vi "prova1.vi"() -> ()   [LabVIEW 2020]
uses:
  <vilib>/Analysis/6fits.llb/Confidence Interval (Linear).vi
  <vilib>/Utility/file.llb/Write Delimited Spreadsheet (DBL).vi
  <vilib>/Analysis/NI_AALPro.lvlib
panel:
  out "delta R (Ohm)":dbl
  out "R (Ohm)":dbl
  out "delta q":dbl
  out "q":dbl
  out "delta m":dbl
  out "m":dbl
  out "Fit i-V":cluster{dbl[], dbl[]}[](graph)
  out "i-V":cluster{dbl[], dbl[]}(graph)
  in  "Device Name":tag
  in  "N step":dbl
  in  "Vmin":dbl
  in  "Vmax":dbl
  in  "Esci":bool
  in  "Salva Dati":bool
  in  "Misura":bool
  in  "Analizza":bool
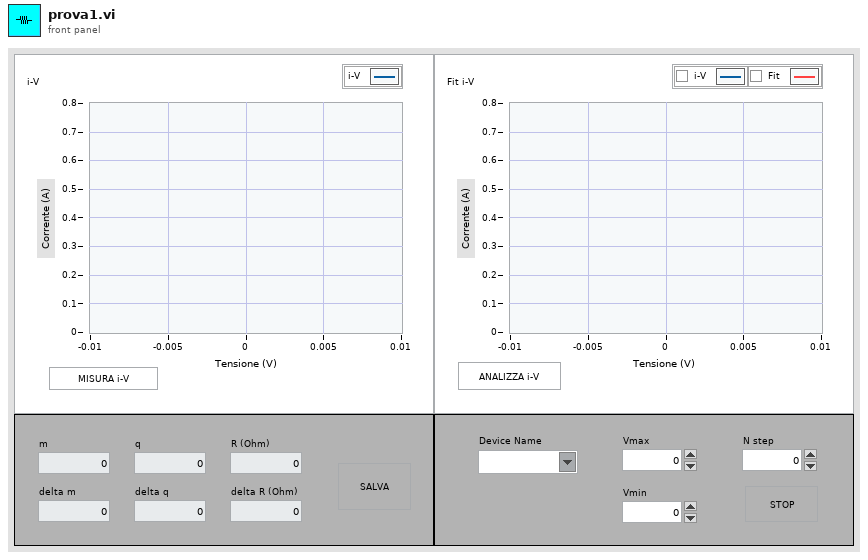
[diagram p1: front panel]
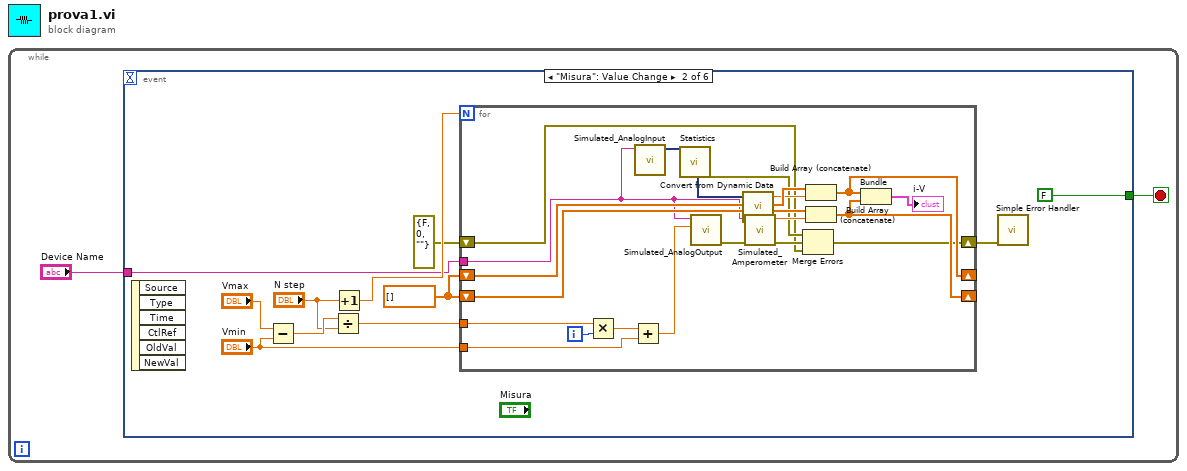
[diagram p0: block diagram]
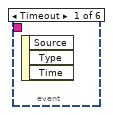
[diagram p2: hidden frame]
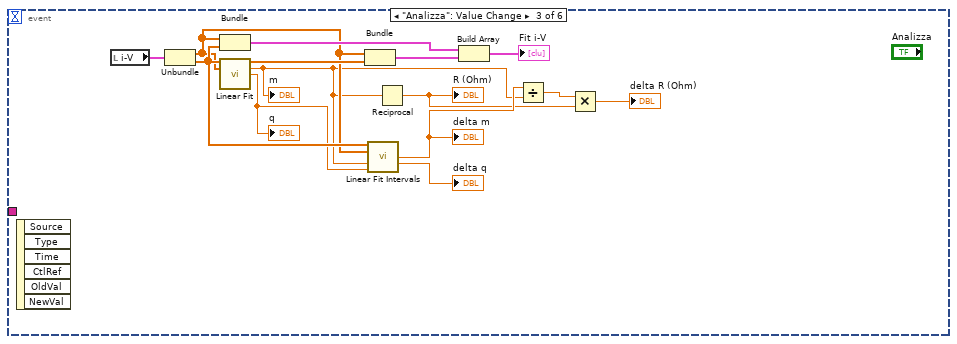
[diagram p3: hidden frame]
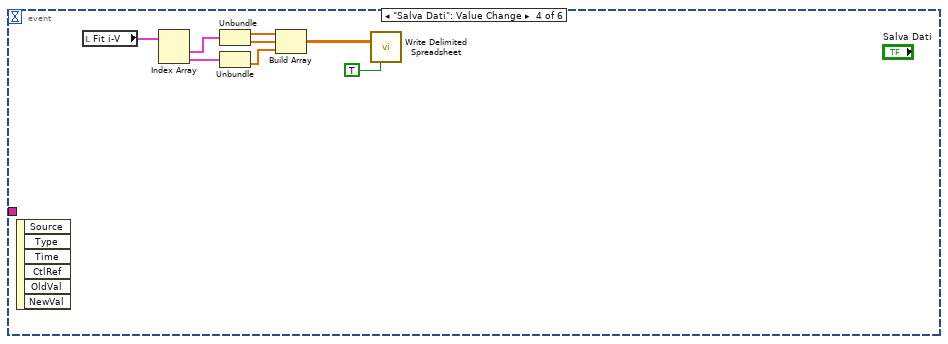
[diagram p4: hidden frame]
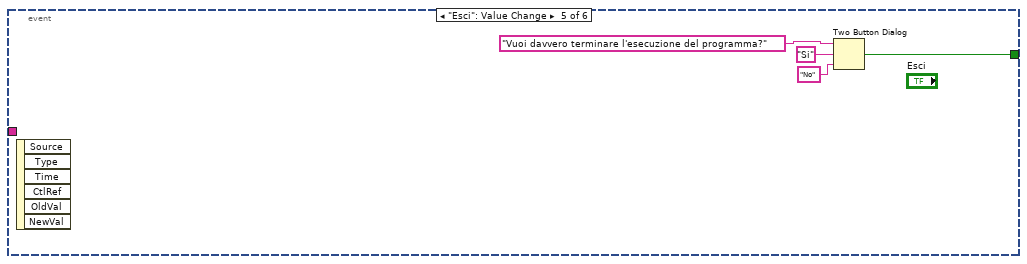
[diagram p5: hidden frame]
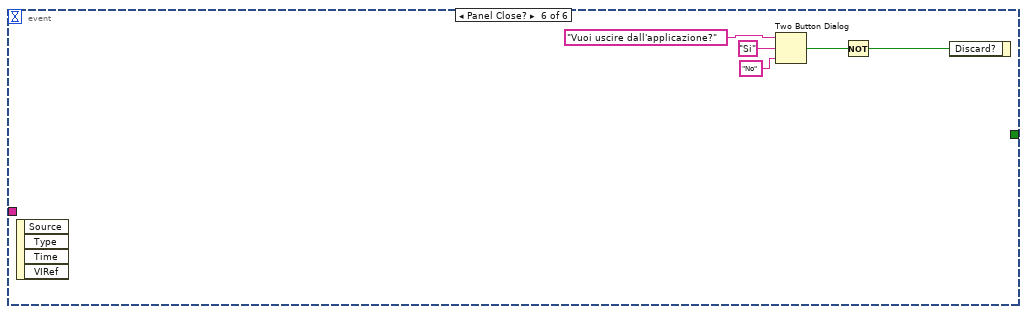
[diagram p6: hidden frame]
diagram:
  n1 = while {
    stop <- w2 stop-if-true
    n2 = event shown="[1] \"Misura\": Value Change" {
      selector: _ -> [_ _ _ _ _ _]
      dyn-events: _ -> [_ _ _ _ _ _]
      timeout: _ -> [_ _ _ _ _ _]
      tunnel: [_ FALSE _ _ w56 _] -> w2
      tunnel: "Device Name" -> [_ w6 _ _ _ _]
      event Timeout {
        n3 = event-data() -> ()  [unwired: 1 in, 3 out]
      }
      event "Misura": Value Change {
        w5 = dbl[] []
        n4 = event-data() -> ()  [unwired: 1 in, 6 out]
        n5 = Subtract(x="Vmax", y="Vmin") -> (x-y=w11:dbl)
        n6 = Divide(x=w11, y="N step") -> (x/y=w9:dbl)
        n7 = Increment(x="N step") -> (x+1=w7:dbl)
        n8 = for {
          N: w7 -> [_]
          tunnel: "Vmin" -> [w16]
          tunnel: w9 -> [w33]
          tunnel: w6 -> [w19]
          shift-right: [w24] -> _
          shift-left: w5 -> [w27]
          shift-right: [w25] -> _
          shift-left: w5 -> [w29]
          shift-right: [w17] -> w3
          shift-left: errorcluster {"status"=FALSE, "code"=0, "source"=""} ("error constant") -> [w18]
          i -> [w32]
          n9 = Multiply(x=w33, y=w32) -> (x*y=w15:dbl)
          n10 = Add(x=w15, y=w16) -> (x+y=w14:dbl)
          n11 = call "Simulated_AnalogInput.vi"("Device Name"=w19) -> ("data"=w22:dynamicdata)  [unwired: 9 in, 1 out]
          n12 = call "Statistics"("Signals"=w22) -> ("Arithmetic Mean"=w21:dynamicdata, "error out"=w20:errorcluster)  [unwired: 25 in]
          n13 = call "Simulated_AnalogOutput.vi"("data"=w14, "Device Name"=w19) -> ("error out"=w30:errorcluster)  [unwired: 9 in]
          n14 = call "Convert from Dynamic Data"("Dynamic Data Type"=w21) -> ("Scalar"=w28:dbl)  [unwired: 3 in]
          n15 = call "Simulated_Amperometer.vi"("error in (no error)"=w30, "Device Name"=w19) -> ("error out"=w31:errorcluster, "Measurement"=w26:dbl)  [unwired: 8 in]
          n16 = Merge Errors(w20, w31, w18) -> (w17:errorcluster)
          n17 = Build Array (concatenate)(w29, w28) -> (w25:dbl[])
          n18 = Build Array (concatenate)(w27, w26) -> (w24:dbl[])
          n19 = Bundle(w25, w24) -> (→"i-V":cluster{dbl[], dbl[]})  [unwired: 1 in]
        }
        n20 = call <vilib>:"Simple Error Handler.vi"("error in (no error)"=w3) -> ()  [unwired: 4 in, 5 out]
      }
      event "Analizza": Value Change {
        n21 = event-data() -> ()  [unwired: 1 in, 6 out]
        n22 = local read "i-V"() -> (w47:cluster{dbl[], dbl[]})
        n23 = Unbundle(w47) -> (w41:dbl[], w43:dbl[])
        n24 = Bundle(w41, w43) -> (w46:cluster{dbl[], dbl[]})  [unwired: 1 in]
        n25 = call <vilib>:"Linear Fit.vi"("Y"=w43, "X"=w41) -> ("Best Linear Fit"=w42:dbl[], "slope"=w37:dbl, "intercept"=w39:dbl)  [unwired: 9 in, 2 out]
        "q" <- w39
        "m" <- w37
        n26 = Bundle(w41, "Best Linear Fit"=w42) -> (w45:cluster{dbl[], "Best Linear Fit":dbl[]})  [unwired: 1 in]
        n27 = call-poly <vilib>:"Linear Fit Intervals.vi"("Y"=w43, "X"=w41, "slope"=w37, "intercept"=w39) -> ("delta slope"=w38:dbl, "delta intercept"=→"delta q":dbl)  [unwired: 7 in, 3 out]
        "delta m" <- w38
        n28 = Reciprocal(x=w37) -> (1/x=w34:dbl)
        "R (Ohm)" <- w34
        n29 = Build Array(w46, w45) -> (→"Fit i-V":cluster{dbl[], "Best Linear Fit":dbl[]}[])
        n30 = Divide(x=w38, y=w37) -> (x/y=w36:dbl)
        n31 = Multiply(x=w36, y=w34) -> (x*y=→"delta R (Ohm)":dbl)
      }
      event "Salva Dati": Value Change {
        n32 = event-data() -> ()  [unwired: 1 in, 6 out]
        n33 = local read "Fit i-V"() -> (w55:cluster{dbl[], dbl[]}[])
        n34 = Index Array(array=w55) -> (element #1=w54:cluster{dbl[], dbl[]}, element #2=w53:cluster{dbl[], dbl[]})  [unwired: 2 in]
        n35 = Unbundle(w54) -> (w52:dbl[], w51:dbl[])
        n36 = Unbundle(w53) -> (w50:dbl[])  [unwired: 1 out]
        n37 = Build Array(w52, w51, w50) -> (w48:dbl[][])
        n38 = call-poly <vilib>:"Write Delimited Spreadsheet.vi"("2D data"=w48, "transpose? (no:F)"=TRUE) -> ()  [unwired: 12 in, 2 out]
      }
      event "Esci": Value Change {
        n39 = event-data() -> ()  [unwired: 1 in, 6 out]
        n40 = Two Button Dialog(message="Vuoi davvero terminare l'esecuzione del programma?", 1:"No", 2:"Si") -> (T button?=w56:bool)
      }
      event Panel Close? {
        n41 = event-data() -> ()  [unwired: 1 in, 4 out]
        n42 = Two Button Dialog(message="Vuoi uscire dall'applicazione?", 1:"No", 2:"Si") -> (T button?=w61:bool)
        n43 = Not(x=w61) -> (.not. x?=w60:bool)
        n44 = event-data("Discard?"=w60) -> ()  [unwired: 1 in, 1 out]
      }
    }
  }
